vi "DSF.Engine.Runtime.Plugin.Wait for Transfer Group.vi"(8 "error in (no error)":errorcluster, 11 "Plugin Runtime in":refnum<class "DSF.Engine.Runtime.Plugin.lvclass">) -> (0 "error out":errorcluster, 3 "Plugin Runtime out":refnum<class "DSF.Engine.Runtime.Plugin.lvclass">)   [LabVIEW 2016, in "DSF.Engine.lvlib" / "DSF.Engine.Runtime.Plugin.lvclass"]
uses:
  DSF.Engine.Runtime.Plugin.lvclass
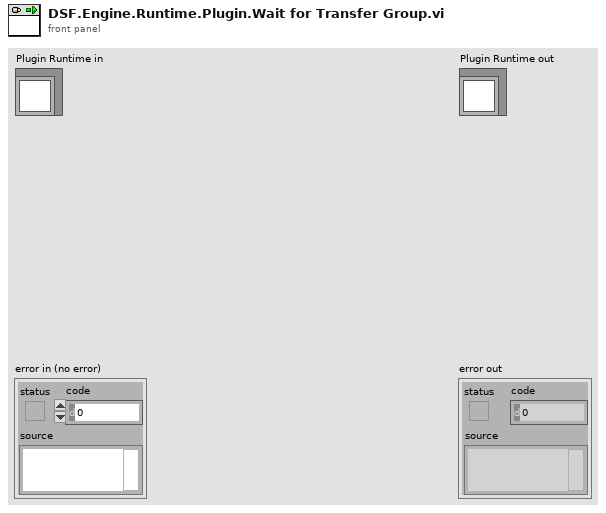
[diagram p1: front panel]
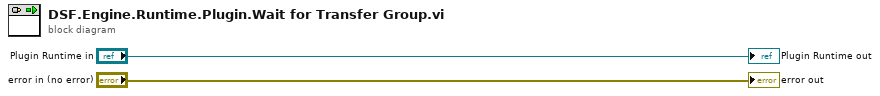
[diagram p0: block diagram]
diagram:
  "error out" <- "error in (no error)"
  "Plugin Runtime out" <- "Plugin Runtime in"
